vi "Main.vi"() -> ()   [LabVIEW 2022 SP3]
doc: "This template is for the Queued Message Handler design pattern.\n\nThe Event Handling Loop generates messages based on user interface actions.\n\nThe Message Handling Loop processes messages generated by the Event Handling Loop, or by other messages. The messages are string values, so new messages can be added easily to the Message Cases case structure in the Message Handling Loop. Each message cluster can also provide an optional value for Message Data, which is a variant that can be converted to whatever message-specific data is required."
uses:
  controls/MHL Data.ctl
  controls/MHL UI Data.ctl
  controls/MHL Status.ctl
  controls/MHL References.ctl
  controls/MHL Configuration.ctl
  support/Boiler System Globals.vi
  support/Message Queue/Message Queue.lvlib
  support/User Event - Stop/User Event - Stop.lvlib
  Boiler/Boiler.lvlib
panel:
  out "Forced Draft Fan":bool
  out "Pilot":bool
  out "Pilot Gas Valve":bool
  out "Primary Fan":bool
  out "Status":string
  in  "Fuel Control Valve":u32(slide) scale=10.0..75.0
  in  "Emergency Stop":bool
  in  "Stop Boiler":bool
  in  "Light Pilot":bool
  in  "Start":bool
  in  "Reset":bool
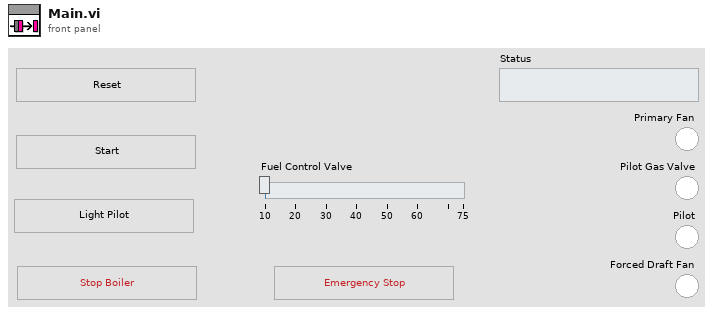
[diagram p1: front panel]
types:
  T1 = typedef "MHL Data.ctl" = cluster{"MHL User Interface Data":T2, "MHL References":T4, "MHL Configuration":T5}
  T2 = typedef "MHL UI Data.ctl" = cluster{"Status":string, "Fuel Control Valve":u32, "Primary Fan":bool, "Pilot Gas Valve":bool, "Pilot":bool, "Forced Draft Fan":bool, "MHL Status":T3}
  T3 = typedef "MHL Status.ctl" = enum16{"Lockout", "Ready", "Pre-Purge", "Pre-Purge Complete", "Pilot On", "Boiler Running", "Shutdown", "Purge"}
  T4 = typedef "MHL References.ctl" = cluster{"Reset Ref":refnum<vi>, "Start Ref":refnum<vi>, "Light Pilot Ref":refnum<vi>, "Stop Boiler Ref":refnum<vi>, "Fuel Control Valve Ref":refnum<vi>}
  T5 = typedef "MHL Configuration.ctl" = cluster{"Fuel Control Valve Maximum":dbl, "Fuel Control Valve Minimum":dbl}
  T6 = typedef "Notifiers.ctl" = cluster{"Handshake":refnum<notifier>, "Flame Level":refnum<notifier>, "Controller Exit":refnum<notifier>, "Boiler Ext":refnum<notifier>}
  T7 = typedef "Message Queue.lvlib/All Message Queues.ctl" = cluster{"MHL":refnum<queue>, "Boiler Controller":refnum<queue>, "Boiler":refnum<queue>}
  T8 = enum32{"invalid app kind", "Development System", "Run Time System", "Student Edition", "Embedded LabVIEW", "Evaluation", "Custom"}
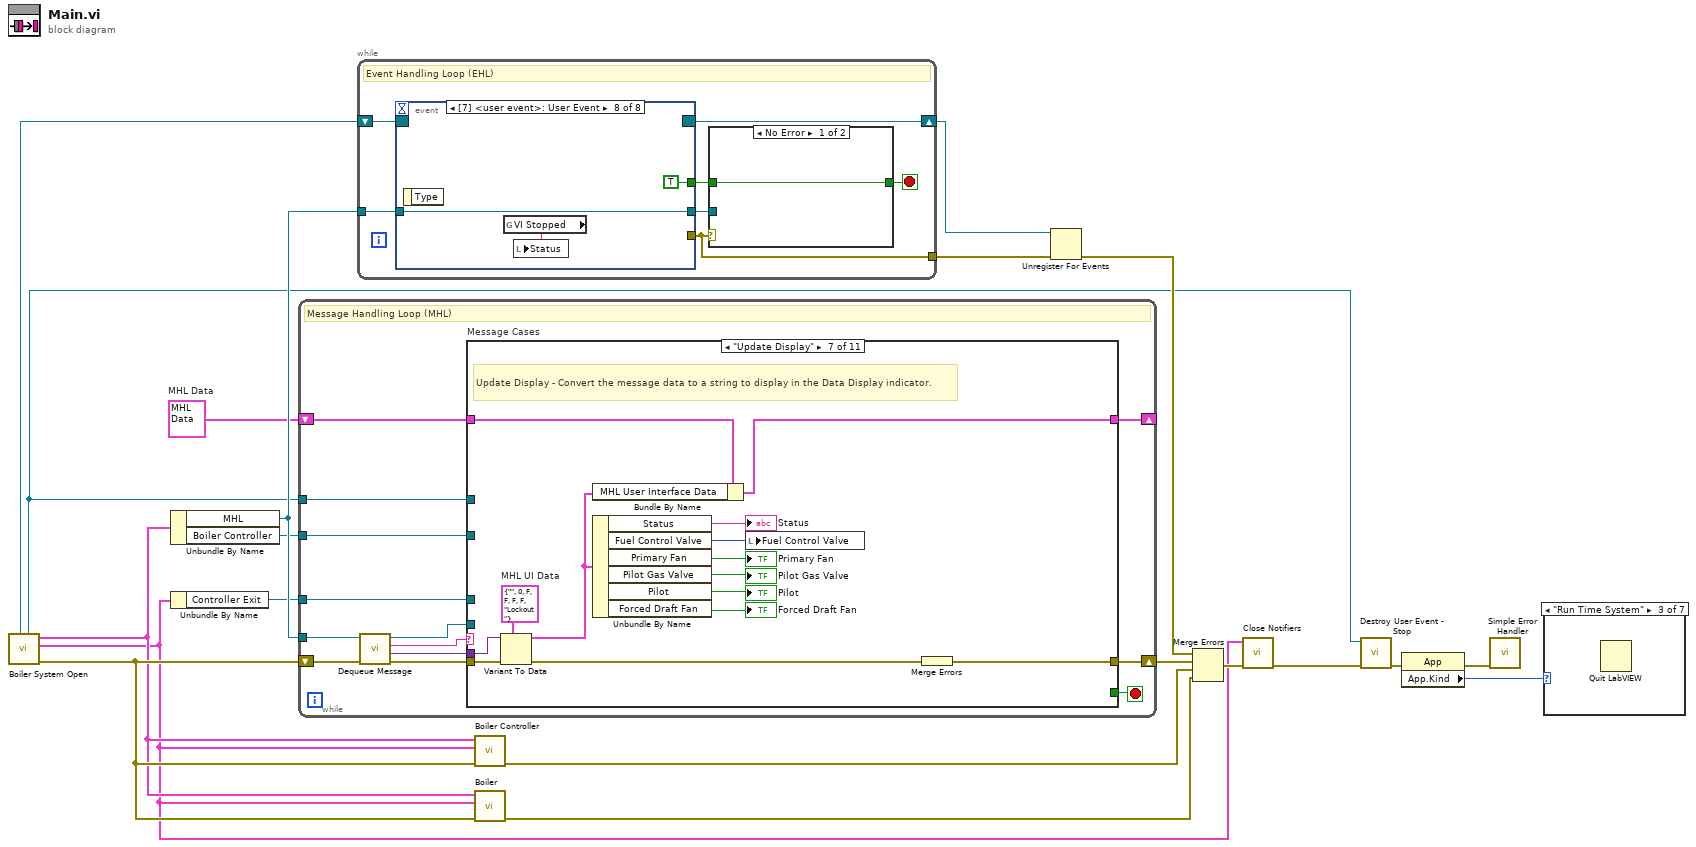
[diagram p0: block diagram]
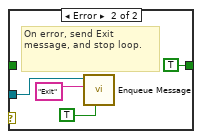
[diagram p8: hidden frame]
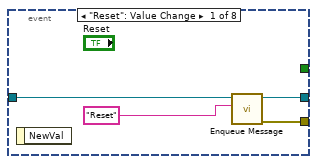
[diagram p9: hidden frame]
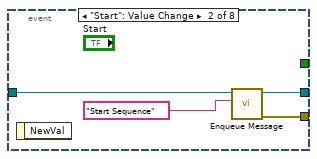
[diagram p10: hidden frame]
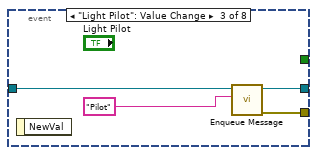
[diagram p11: hidden frame]
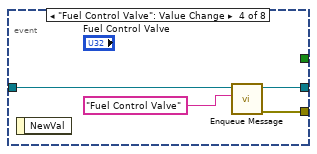
[diagram p12: hidden frame]
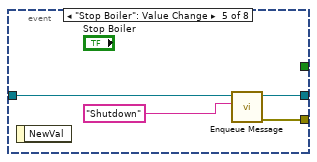
[diagram p13: hidden frame]
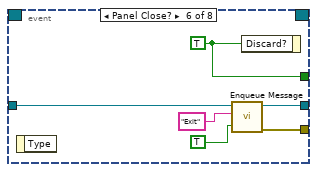
[diagram p14: hidden frame]
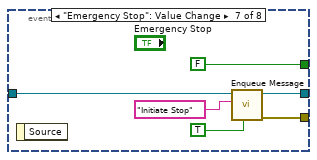
[diagram p15: hidden frame]
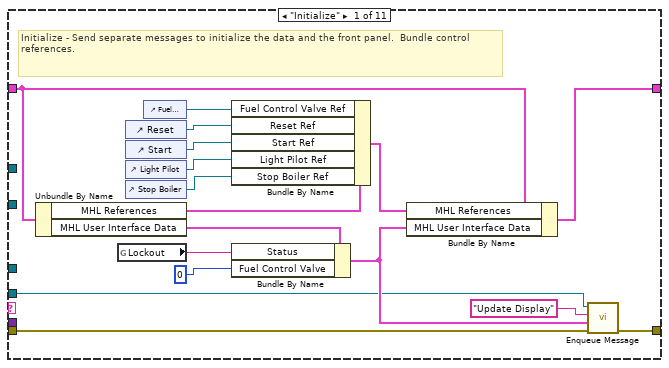
[diagram p16: hidden frame]
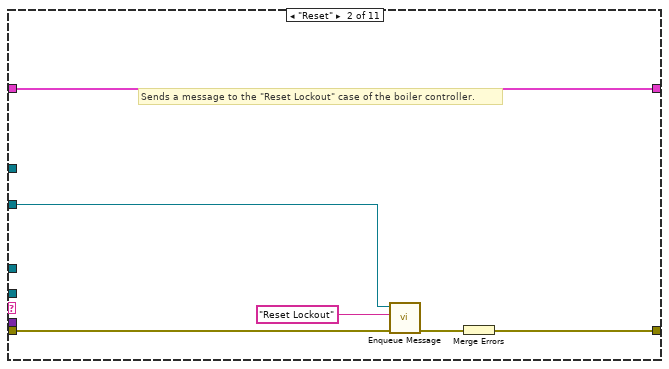
[diagram p17: hidden frame]
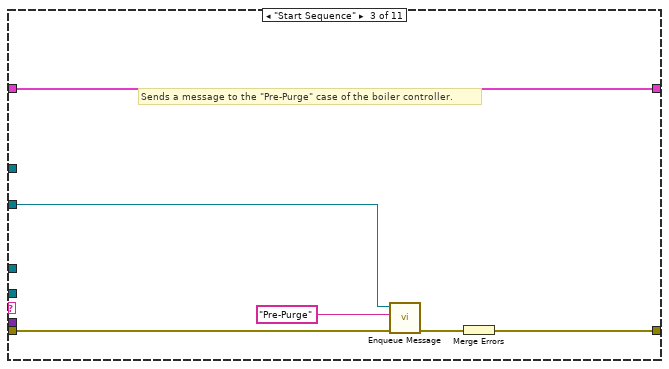
[diagram p18: hidden frame]
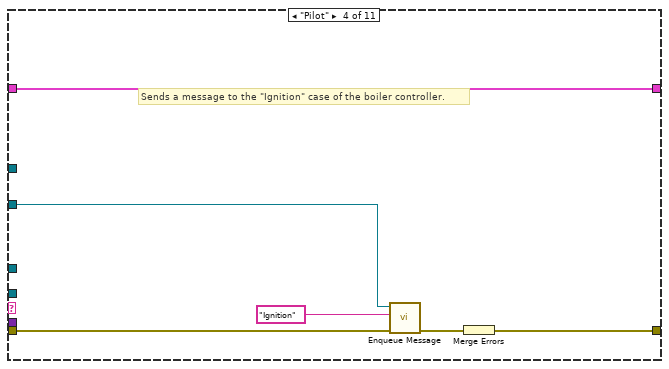
[diagram p19: hidden frame]
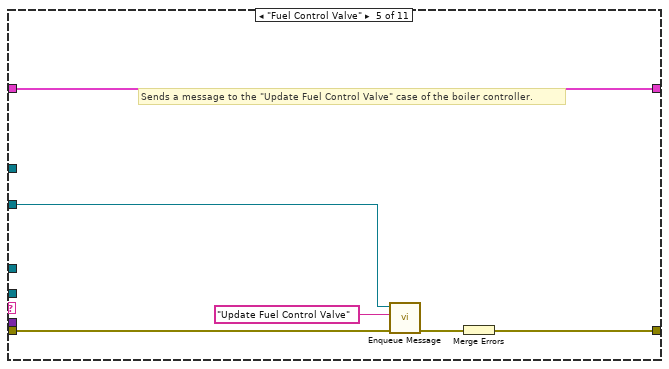
[diagram p20: hidden frame]
diagram:
  w1 = T1 {"MHL User Interface Data"={"Status"="", "Fuel Control Valve"=0, "Primary Fan"=FALSE, "Pilot Gas Valve"=FALSE, "Pilot"=FALSE, "Forced Draft Fan"=FALSE, "MHL Status"=enum."Lockout"}, "MHL References"={"Reset Ref"=refnum, "Start Ref"=refnum, "Light Pilot Ref"=refnum, "Stop Boiler Ref"=refnum, "Fuel Control Valve Ref"=refnum}, "MHL Configuration"={"Fuel Control Valve Maximum"=0.0, "Fuel Control Valve Minimum"=0.0}}  # MHL Data
  n1 = call "Boiler System Open.vi"() -> ("error out"=w8:errorcluster, "Notifiers"=w3:T6, "Message Queues"=w7:T7, "User Event - Stop"=w9:refnum<user-event>, "Stop Event Registration Refnum"=w10:refnum<event-registration>)  [unwired: 7 in]
  n2 = Unbundle By Name(w7) -> ("MHL"=w19:refnum<queue>, "Boiler Controller"=w15:refnum<queue>)
  n3 = Unbundle By Name(w3) -> ("Controller Exit"=w6:refnum<notifier>)
  n4 = while {
    tunnel: w19 -> [w23]
    shift-right: [w32] -> _
    shift-left: w1 -> [w33]
    tunnel: w9 -> [w29]
    shift-right: [w30] -> w20
    shift-left: w8 -> [w28]
    tunnel: w15 -> [w22]
    tunnel: w6 -> [w21]
    stop <- w31 stop-if-true
    # "Message Handling Loop (MHL)"
    n5 = call "Dequeue Message.vi"("error in"=w28, "Message Queue"=w23) -> ("error out"=w27:errorcluster, "Message Data"=w25:variant, "Message"=w26:string, "dup Message Queue"=w24:refnum<queue>)  [unwired: 6 in]
    n6 = case "Message Cases" shown="\"Update Display\"" w26 {
      selector: w26 -> [_ _ _ _ _ _ _ _ _ _ w130]
      tunnel: w24 -> [w34 _ _ _ _ _ _ w96 w112 w126 _]
      tunnel: w27 -> [w36 w54 w60 w66 w72 w78 w93 w101 w117 w121 _]
      tunnel: [w50 w55 w61 w67 w73 w79 w94 w95 w115 w122 w128] -> w30
      tunnel: w33 -> [w39 w56 w62 w68 w74 w80 w89 w102 w118 w125 w132]
      tunnel: [w37 w56 w62 w68 w74 w80 w82 w102 w118 w125 w132] -> w32
      tunnel: [_ _ _ _ _ _ _ _ _ TRUE _] -> w31
      tunnel: w25 -> [_ _ _ _ _ _ w92 _ _ _ _]
      tunnel: w29 -> [_ _ _ _ _ _ _ _ _ w120 _]
      tunnel: w22 -> [_ w51 w57 w63 w69 w75 _ _ w111 _ _]
      tunnel: w21 -> [_ _ _ _ _ _ _ w100 _ _ _]
      frame "Initialize" {
        # "Initialize - Send separate messages to initialize the data and the front panel.  Bundle control references."
        n7 = Unbundle By Name(w39) -> ("MHL References"=w48:T4, "MHL User Interface Data"=w47:T2)
        n8 = global read "Boiler System Globals.vi" "Lockout"() -> (w46:string)
        n9 = control-ref of="Reset"() -> (w43:refnum<vi>)
        n10 = control-ref of="Start"() -> (w42:refnum<vi>)
        n11 = control-ref of="Light Pilot"() -> (w41:refnum<vi>)
        n12 = control-ref of="Stop Boiler"() -> (w40:refnum<vi>)
        n13 = control-ref of="Fuel Control Valve"() -> (w44:refnum<vi>)
        n14 = Bundle By Name(cluster=w48, "Fuel Control Valve Ref"=w44, "Reset Ref"=w43, "Start Ref"=w42, "Light Pilot Ref"=w41, "Stop Boiler Ref"=w40) -> (w38:T4)
        n15 = Bundle By Name(cluster=w47, "Status"=w46, "Fuel Control Valve"=u32 0) -> (w35:T2)
        n16 = Bundle By Name(cluster=w39, "MHL References"=w38, "MHL User Interface Data"=w35) -> (w37:T1)
        n17 = call "Enqueue Message.vi"("error in"=w36, "Message Data"=w35, "Message"="Update Display", "Message Queue"=w34) -> ("error out"=w50:errorcluster)  [unwired: 6 in, 1 out]
      }
      frame "Reset" {
        # "Sends a message to the \"Reset Lockout\" case of the boiler controller."
        n18 = call "Enqueue Message.vi"("error in"=w54, "Message"="Reset Lockout", "Message Queue"=w51) -> ("error out"=w53:errorcluster)  [unwired: 7 in, 1 out]
        n19 = Merge Errors(w53) -> (w55:errorcluster)
      }
      frame "Start Sequence" {
        # "Sends a message to the \"Pre-Purge\" case of the boiler controller."
        n20 = call "Enqueue Message.vi"("error in"=w60, "Message"="Pre-Purge", "Message Queue"=w57) -> ("error out"=w59:errorcluster)  [unwired: 7 in, 1 out]
        n21 = Merge Errors(w59) -> (w61:errorcluster)
      }
      frame "Pilot" {
        # "Sends a message to the \"Ignition\" case of the boiler controller."
        n22 = call "Enqueue Message.vi"("error in"=w66, "Message"="Ignition", "Message Queue"=w63) -> ("error out"=w65:errorcluster)  [unwired: 7 in, 1 out]
        n23 = Merge Errors(w65) -> (w67:errorcluster)
      }
      frame "Fuel Control Valve" {
        # "Sends a message to the \"Update Fuel Control Valve\" case of the boiler controller."
        n24 = call "Enqueue Message.vi"("error in"=w72, "Message"="Update Fuel Control Valve", "Message Queue"=w69) -> ("error out"=w71:errorcluster)  [unwired: 7 in, 1 out]
        n25 = Merge Errors(w71) -> (w73:errorcluster)
      }
      frame "Shutdown" {
        # "Sends a message to the \"Shutdown\" case of the boiler controller."
        n26 = call "Enqueue Message.vi"("error in"=w78, "Message"="Shutdown", "Message Queue"=w75) -> ("error out"=w77:errorcluster)  [unwired: 7 in, 1 out]
        n27 = Merge Errors(w77) -> (w79:errorcluster)
      }
      frame "Update Display" {
        w90 = T2 {"Status"="", "Fuel Control Valve"=0, "Primary Fan"=FALSE, "Pilot Gas Valve"=FALSE, "Pilot"=FALSE, "Forced Draft Fan"=FALSE, "MHL Status"=enum."Lockout"}  # MHL UI Data
        # "Update Display - Convert the message data to a string to display in the Data Display indicator."
        n28 = Variant To Data(error in=w93, type=w90, Variant=w92) -> (data=w81:T2, error out=w91:errorcluster)
        n29 = Bundle By Name(cluster=w89, "MHL User Interface Data"=w81) -> (w82:T1)
        n30 = Unbundle By Name(w81) -> ("Status"=→"Status":string, "Fuel Control Valve"=w87:u32, "Primary Fan"=→"Primary Fan":bool, "Pilot Gas Valve"=→"Pilot Gas Valve":bool, "Pilot"=→"Pilot":bool, "Forced Draft Fan"=→"Forced Draft Fan":bool)
        n31 = local write "Fuel Control Valve"(w87) -> ()
        n32 = Merge Errors(w91) -> (w94:errorcluster)
      }
      frame "Wait on Boiler Exit" {
        n33 = Wait on Notification(notifier=w100, timeout in ms (-1)=10, error in (no error)=w101) -> (timed out?=w97:bool, error out=w98:errorcluster)  [unwired: 1 in, 2 out]
        n34 = case shown="False" w97 {
          tunnel: w98 -> [w105 w110]
          tunnel: w96 -> [w104 w109]
          tunnel: [w106 w108] -> w95
          frame False {
            n35 = call "Enqueue Message.vi"("error in"=w105, "Message"="Exit", "Message Queue"=w104) -> ("error out"=w106:errorcluster)  [unwired: 7 in, 1 out]
          }
          frame True {
            n36 = call "Enqueue Message.vi"("error in"=w110, "Message"="Wait on Boiler Exit", "Message Queue"=w109) -> ("error out"=w108:errorcluster)  [unwired: 7 in, 1 out]
          }
        }
      }
      frame "Initiate Stop" {
        # "When stopping, first send a message to stop the boiler controller.\nThen wait for the boiler and boiler controller to ext"
        n37 = call "Enqueue Message.vi"("error in"=w117, "Message"="Exit", "Message Queue"=w111) -> ("error out"=w116:errorcluster)  [unwired: 7 in, 1 out]
        n38 = call "Enqueue Message.vi"("error in"=w116, "Message"="Wait on Boiler Exit", "Message Queue"=w112) -> ("error out"=w115:errorcluster)  [unwired: 7 in, 1 out]
      }
      frame "Exit" {
        # "Stop the VI"
        # "Release the message queue reference"
        n39 = call "Fire User Event - Stop.vi"("User Event - Stop"=w120) -> ("error out"=w119:errorcluster)  [unwired: 10 in]
        n40 = Release Queue(queue=w126, error in (no error)=w121) -> (error out=w123:errorcluster)  [unwired: 1 in, 2 out]
        n41 = Merge Errors(w119, w123) -> (w122:errorcluster)
      }
      frame Default {
        # "'Default' case only runs if there is a message that isn't defined in any of the other cases.  Output a programming error."
        n42 = Format Into String(format string="The invalid message string \"%s\" was received in the Message Handling Loop." ("Unknown Message Error Text"), w130) -> (resulting string=w127:string)  [unwired: 2 in, 1 out]
        n43 = call <vilib>:"Error Cluster From Error Code.vi"("error message (\"\")"=w127, "error code (0)"=1) -> ("error out"=w128:errorcluster)  [unwired: 7 in]
      }
    }
  }
  n44 = while {
    tunnel: w19 -> [w139]
    tunnel: [w135] -> w17
    shift-right: [w133] -> w16
    shift-left: w10 -> [w134]
    stop <- w137 stop-if-true
    # "Event Handling Loop (EHL)"
    n45 = event shown="[7] <user event>: User Event" {
      selector: w134 -> [_ _ _ _ _ _ _ _]
      dyn-events: [_ _ _ _ _ _ _ _] -> w133
      timeout: _ -> [_ _ _ _ _ _ _ _]
      tunnel: [_ _ _ _ _ w170 FALSE ("Discard?") TRUE ("Discard?")] -> w138
      tunnel: w139 -> [w148 w152 w156 w160 w164 w169 w176 w179]
      tunnel: [w147 w151 w155 w159 w163 w168 w175 _] -> w135
      tunnel: [w146 w150 w154 w158 w162 w167 w173 w179] -> w136
      event "Reset": Value Change {
        n46 = event-data() -> ()  [unwired: 1 in, 1 out]
        n47 = call "Enqueue Message.vi"("Message"="Reset", "Message Queue"=w148) -> ("error out"=w147:errorcluster, "dup Message Queue"=w146:refnum<queue>)  [unwired: 8 in]
      }
      event "Start": Value Change {
        n48 = event-data() -> ()  [unwired: 1 in, 1 out]
        n49 = call "Enqueue Message.vi"("Message"="Start Sequence", "Message Queue"=w152) -> ("error out"=w151:errorcluster, "dup Message Queue"=w150:refnum<queue>)  [unwired: 8 in]
      }
      event "Light Pilot": Value Change {
        n50 = event-data() -> ()  [unwired: 1 in, 1 out]
        n51 = call "Enqueue Message.vi"("Message"="Pilot", "Message Queue"=w156) -> ("error out"=w155:errorcluster, "dup Message Queue"=w154:refnum<queue>)  [unwired: 8 in]
      }
      event "Fuel Control Valve": Value Change {
        n52 = event-data() -> ()  [unwired: 1 in, 1 out]
        n53 = call "Enqueue Message.vi"("Message"="Fuel Control Valve", "Message Queue"=w160) -> ("error out"=w159:errorcluster, "dup Message Queue"=w158:refnum<queue>)  [unwired: 8 in]
      }
      event "Stop Boiler": Value Change {
        n54 = event-data() -> ()  [unwired: 1 in, 1 out]
        n55 = call "Enqueue Message.vi"("Message"="Shutdown", "Message Queue"=w164) -> ("error out"=w163:errorcluster, "dup Message Queue"=w162:refnum<queue>)  [unwired: 8 in]
      }
      event Panel Close? {
        w170 = TRUE ("Discard?")
        n56 = event-data() -> ()  [unwired: 1 in, 1 out]
        n57 = call "Enqueue Message.vi"("Priority Message? (F)"=TRUE, "Message"="Exit", "Message Queue"=w169) -> ("error out"=w168:errorcluster, "dup Message Queue"=w167:refnum<queue>)  [unwired: 7 in]
        n58 = event-data("Discard?"=w170) -> ()  [unwired: 1 in, 1 out]
      }
      event "Emergency Stop": Value Change {
        n59 = event-data() -> ()  [unwired: 1 in, 1 out]
        n60 = call "Enqueue Message.vi"("Priority Message? (F)"=TRUE, "Message"="Initiate Stop", "Message Queue"=w176) -> ("error out"=w175:errorcluster, "dup Message Queue"=w173:refnum<queue>)  [unwired: 7 in]
      }
      event User Event {
        n61 = event-data() -> ()  [unwired: 1 in, 1 out]
        n62 = global read "Boiler System Globals.vi" "VI Stopped"() -> (w177:string)
        n63 = local write "Status"(w177) -> ()
      }
    }
    n64 = case shown="No Error" w135 {
      tunnel: [w140 TRUE ("Discard?")] -> w137
      tunnel: w138 -> [w140 _]
      tunnel: w136 -> [_ w143]
      frame No Error {
      }
      frame Error {
        # "On error, send Exit message, and stop loop."
        n65 = call "Enqueue Message.vi"("Priority Message? (F)"=TRUE, "Message"="Exit", "Message Queue"=w143) -> ()  [unwired: 7 in, 2 out]
      }
    }
  }
  n66 = call "Boiler Controller.vi"("error in"=w8, "Notifiers"=w3, "Message Queues"=w7) -> ("error out"=w14:errorcluster)  [unwired: 8 in]
  n67 = call "Boiler.vi"("error in"=w8, "Notifiers"=w3, "Message Queues"=w7) -> ("error out"=w2:errorcluster)  [unwired: 8 in]
  n68 = Unregister For Events(event registration refnum=w16, error in=w17) -> (error out=w18:errorcluster)
  n69 = Merge Errors(w18, w20, w14, w2) -> (w5:errorcluster)
  n70 = call "Close Notifiers.vi"("error in"=w5, "Notifiers"=w3) -> ("error out"=w4:errorcluster)  [unwired: 9 in]
  n71 = call "Destroy User Event - Stop.vi"("error in"=w4, "User Event - Stop"=w9) -> ("error out"=w13:errorcluster)  [unwired: 9 in]
  n72 = property class="App"(error in=w13) -> (error out=w12:errorcluster, "App.Kind"=w11:T8)  [unwired: 1 in, 1 out]
  n73 = call <vilib>:"Simple Error Handler.vi"("error in (no error)"=w12) -> ()  [unwired: 4 in, 5 out]
  n74 = case shown="\"Run Time System\"" w11 {
    frame "invalid app kind", Default {
    }
    frame "Development System" {
    }
    frame "Run Time System" {
      n75 = Quit LabVIEW() -> ()  [unwired: 1 in]
    }
    frame "Student Edition" {
    }
    frame "Embedded LabVIEW" {
    }
    frame "Evaluation" {
    }
    frame "Custom" {
    }
  }
